vi "一体站流程自动启动.vi"(11 "参数":T1) -> ()   [LabVIEW 2016, in "PLC.lvlib"]
uses:
  PLC.lvlib
panel:
  out "s? t:f":enum16{"初始化", "采配水启动", "仪器操作", "反冲洗", "结束"}(ring)
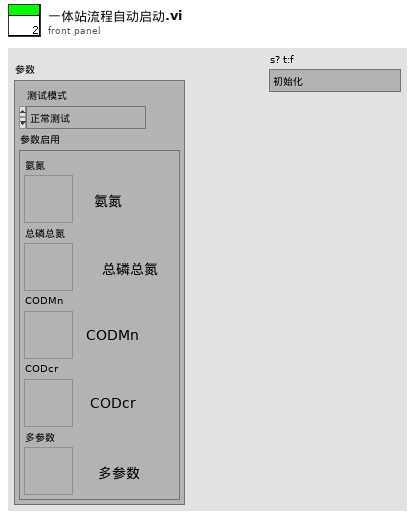
[diagram p1: front panel]
types:
  T1 = cluster{"测试模式":enum16{"正常测试", "集成干预"}, "参数启用":cluster{"氨氮":bool, "总磷总氮":bool, "CODMn":bool, "CODcr":bool, "多参数":bool}}
  T2 = cluster{"命令":string, cluster{"starting address":u16, "holding register value":u16}}
  T3 = enum16{"启动测量", "标样核查", "零点核查", "跨度核查", "空白测试", "平行样测试", "加标回收", "空白校准", "标样校准", "初始化（清洗）", "停止测试", "仪器重启", "校时", "模式设置", "测量间隔设置"}
  T4 = cluster{"时间标识":timestamp, "设备":string, "日志信息":string, "流程参数":string}
  T5 = cluster{"测量模式":enum16{"水样测量", "标样核查", "零点核查", "跨度核查", "空白测试", "加标回收", "平行样", "校零", "校标"}}
  T6 = cluster{"时间标识":timestamp, "设备":string, "日志信息":string}
  T7 = enum16{"空闲", "水样测试", "标样核查", "零点核查", "跨度核查", "空白测试", "平行样测试", "加标回收", "空白校准", "标样校准", "初始化（清洗）"}
  T8 = cluster{"测试时间":dbl, "运行模式":enum16{"维护模式", "常规模式", "应急模式", "质控模式"}}
  T9 = cluster{"R0":i16, "R1":i16, "R2":i16, "R3":i16, "R4":i16, "R5":i16, "R6":i16, "R7":i16, "R8":i16, "R9":i16, "R10":i16, "R11":i16, "R12":i16, "R13":i16, "R14":i16, "R15":i16, "R16":i16, "R17":i16, "R18":i16, "R19":i16, "R20":i16, "R21":i16, "R22":i16, "R23":i16, "R24":i16, "R25":i16, "R26":i16, "R27":i16, "R28":i16, "R29":i16, "R30":i16, "R31":i16, "R32":i16, "R33":i16, "R34":i16}
  T10 = enum32{"Bad", "Idle", "Run top level", "Running"}
  T11 = cluster{"氨氮":bool, "总磷总氮":bool, "CODMn":bool, "CODcr":bool, "多参数":bool}
  T12 = cluster{"水温":dbl, "pH":dbl, "DO":dbl, "Cond":dbl, "Turb":dbl, "叶绿素":dbl, "藻密度":dbl, "蓝绿藻":dbl, "ORP":dbl, "NH3N":dbl}
  T13 = cluster{"时间标识":timestamp, "参数":string, "集成干预测试浓度值":dbl, "集成干预前测试时间":timestamp, "集成干预前测试浓度值":dbl}
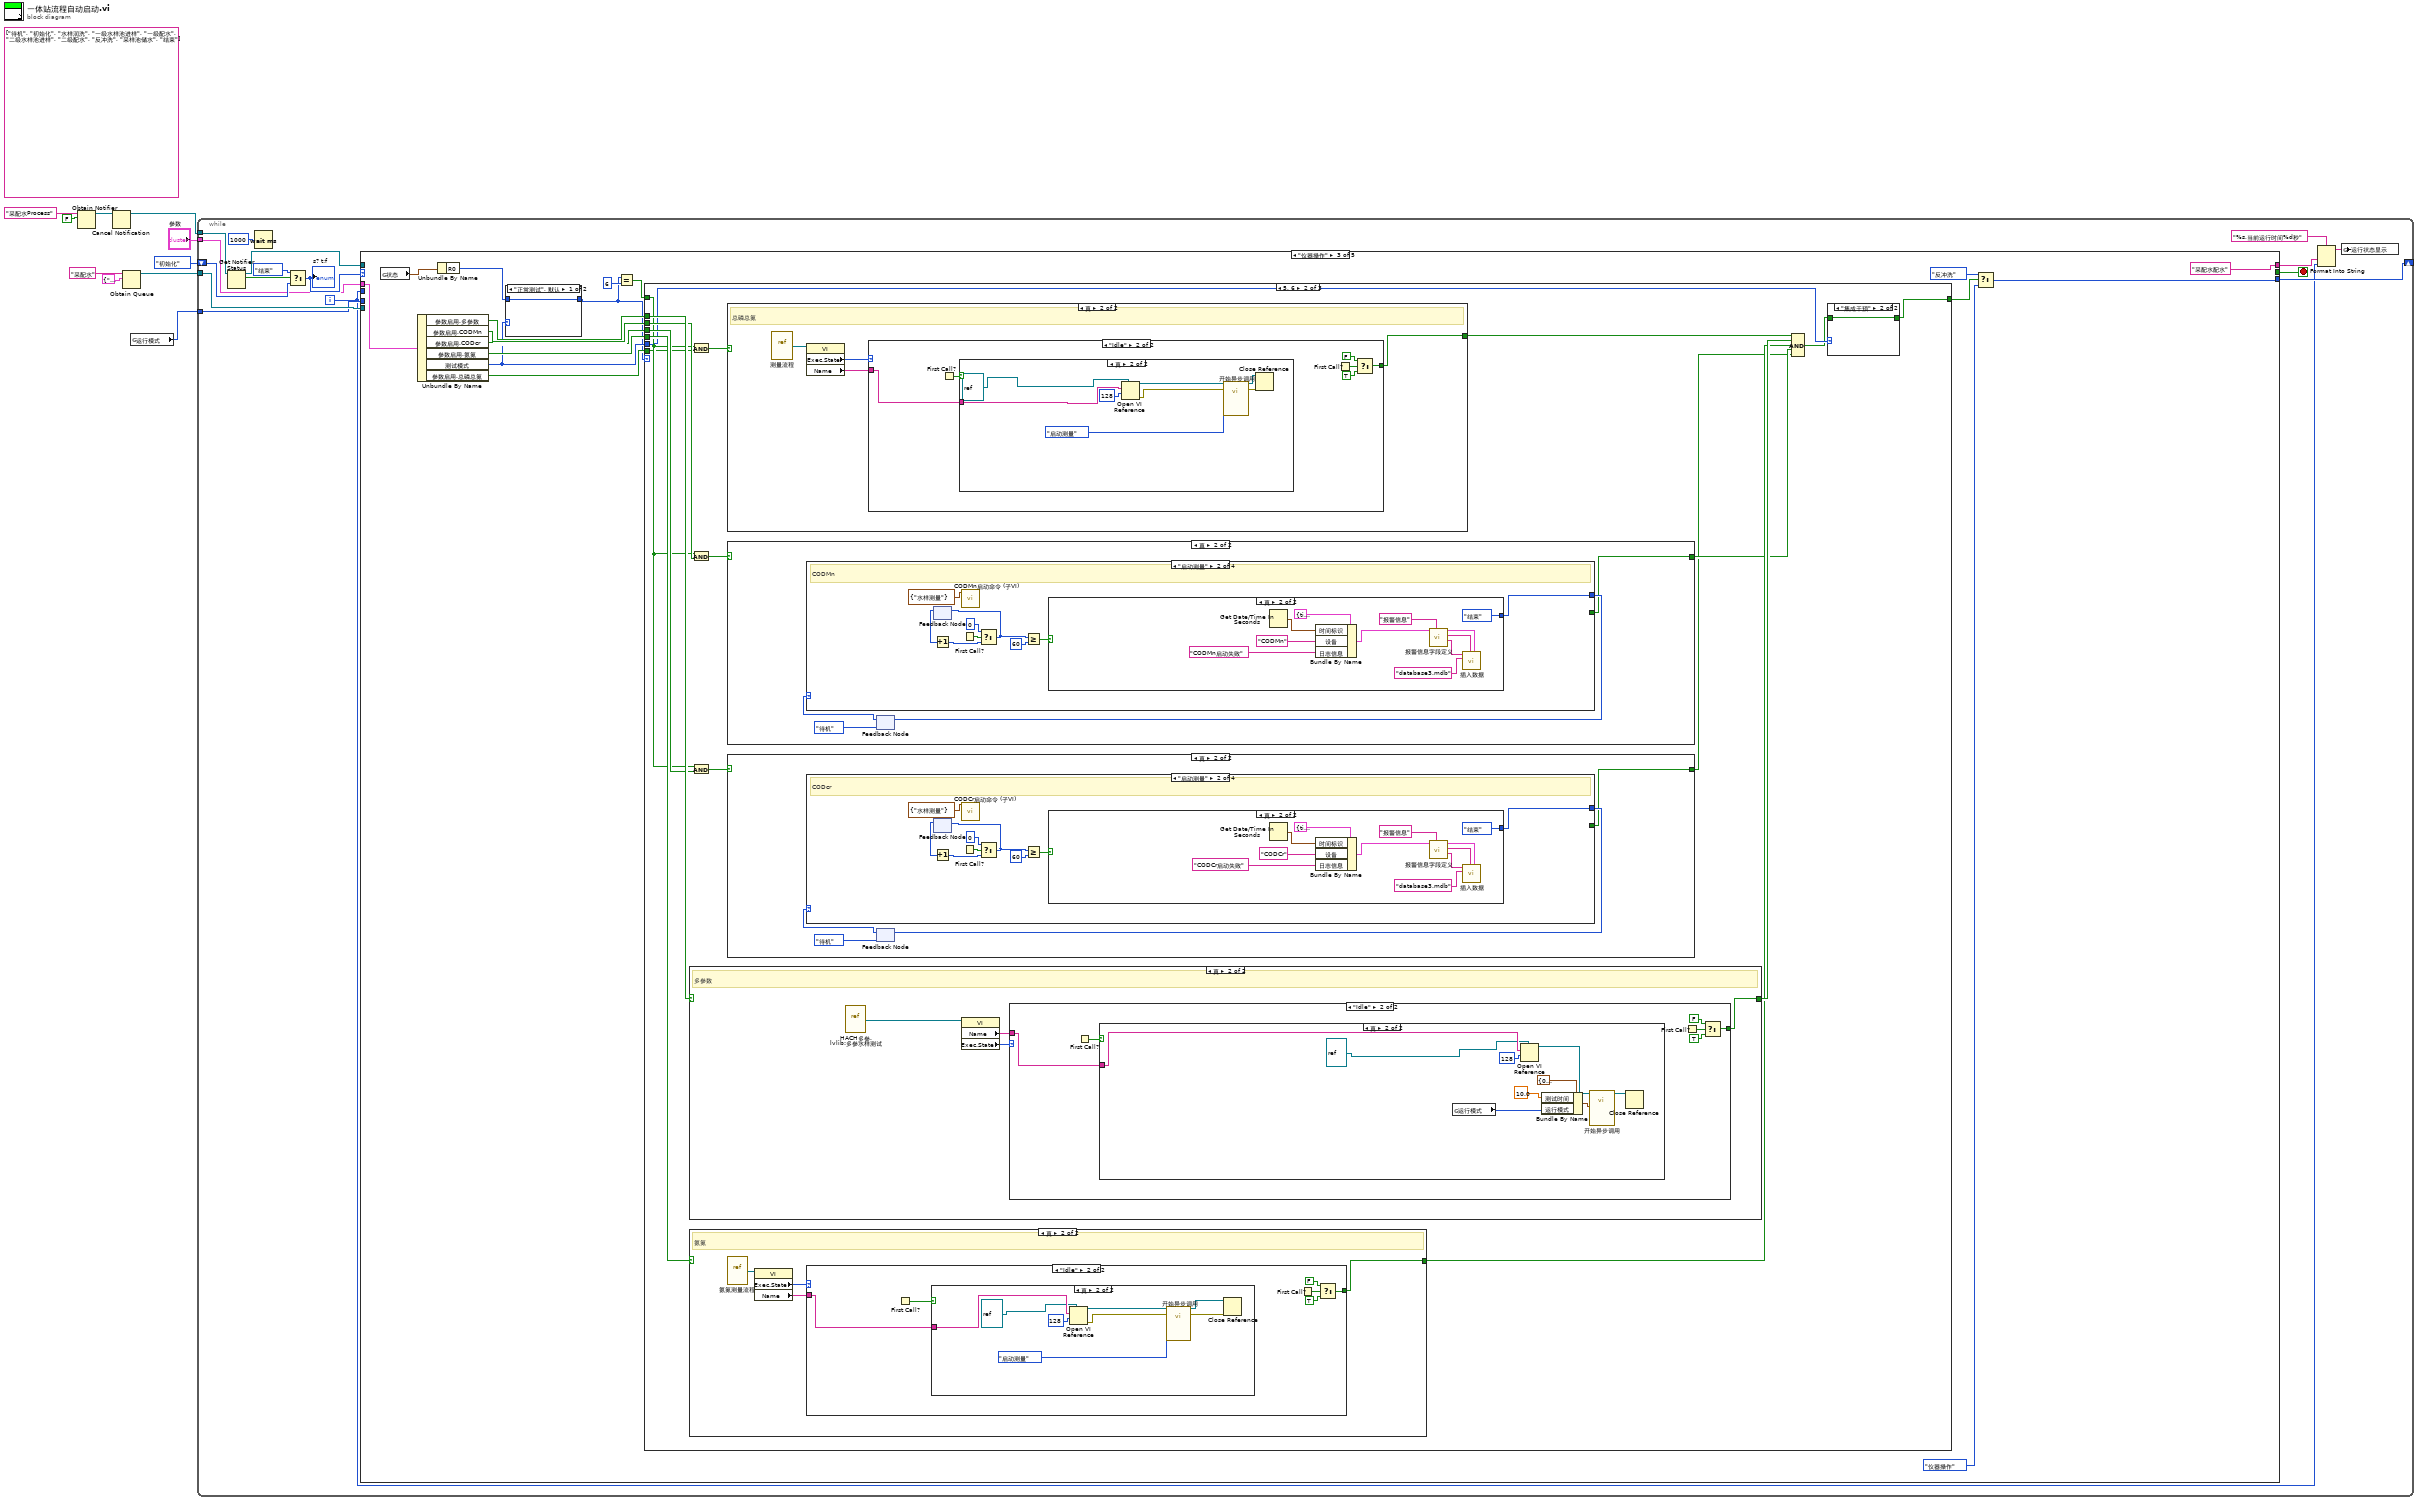
[diagram p0: block diagram]
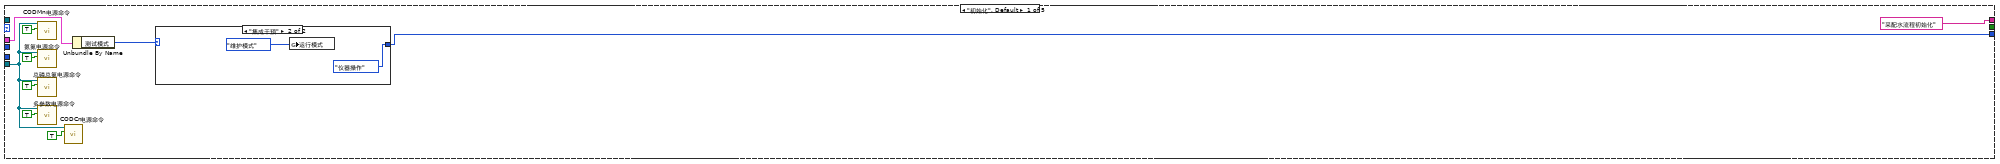
[diagram p2: hidden frame]
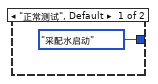
[diagram p3: hidden frame]
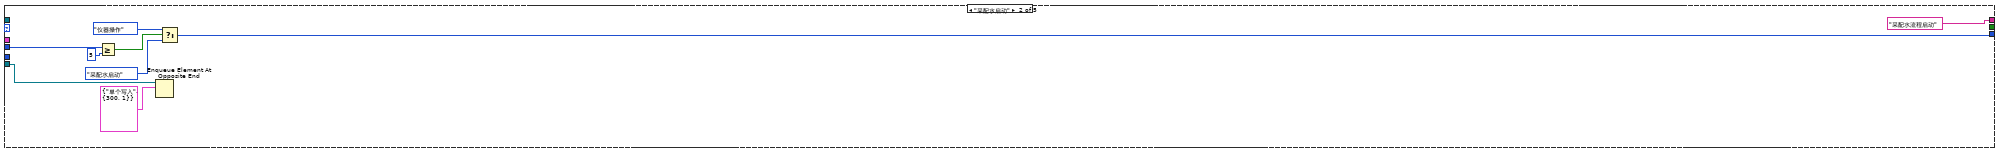
[diagram p4: hidden frame]
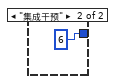
[diagram p5: hidden frame]
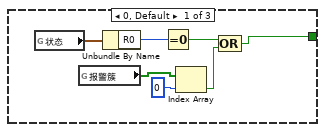
[diagram p6: hidden frame]
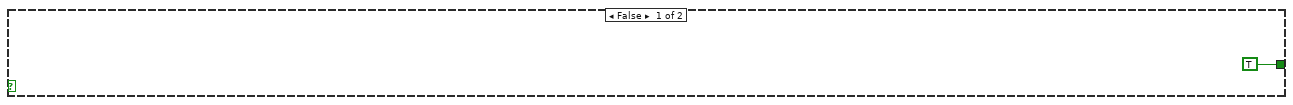
[diagram p7: hidden frame]
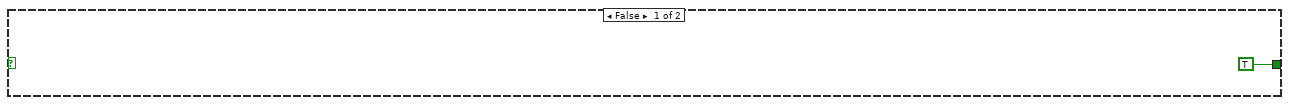
[diagram p11: hidden frame]
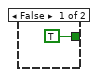
[diagram p14: hidden frame]
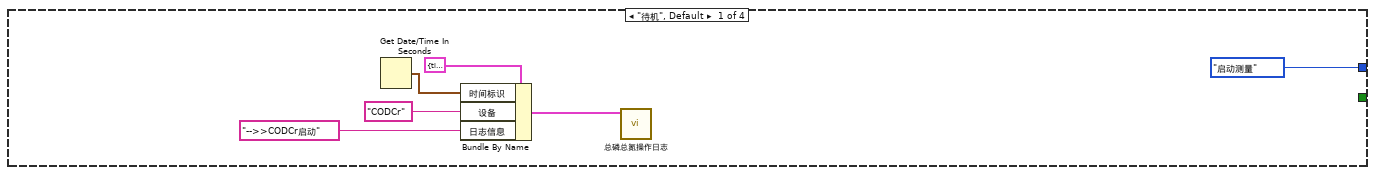
[diagram p15: hidden frame]
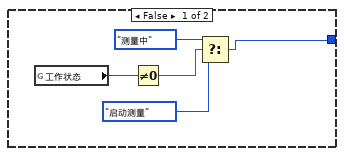
[diagram p16: hidden frame]
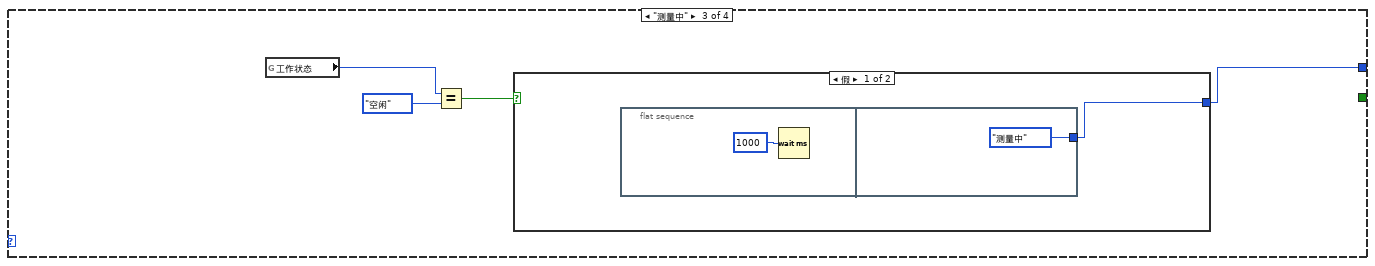
[diagram p17: hidden frame]
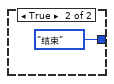
[diagram p18: hidden frame]
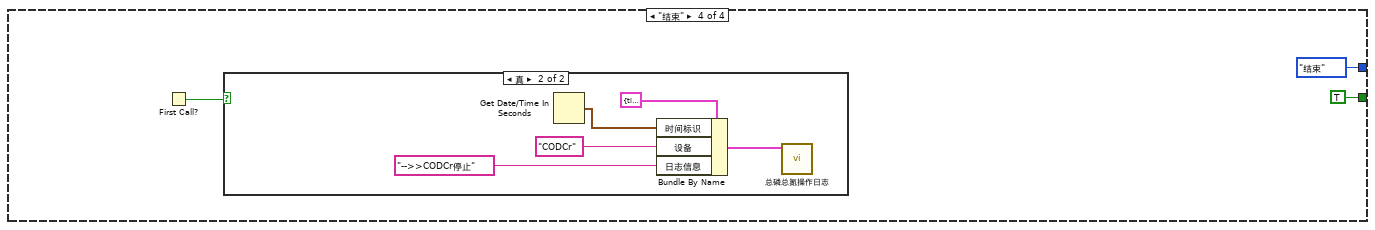
[diagram p19: hidden frame]
diagram:
  (unwired) string[][] [["待机"], ["初始化"], ["水样润洗"], ["一级水样池进样"], ["一级配水"], ["二级水样池进样"], ["二级配水"], ["反冲洗"], ["采样池储水"], ["结束"]] ("项名")
  n1 = Obtain Notifier(name (unnamed)="采配水Process" ("名称（未命名）"), notification data type=FALSE) -> (notifier out=w4:refnum<notifier>)  [unwired: 2 in, 2 out]
  n2 = Cancel Notification(0:w4) -> (8:w3:refnum<notifier>)  [unwired: 1 in, 2 out]
  n3 = Obtain Queue(name (unnamed)="采配水" ("名称（未命名）"), element data type=cluster{"命令":string, "数据":variant} {"命令"="", "数据"=variant}) -> (queue out=w7:refnum<queue>)  [unwired: 3 in, 2 out]
  n4 = global read "系统设置全局变量.vi" "运行模式"() -> (w1:enum16{"维护模式", "常规模式", "应急模式", "质控模式"})
  n5 = while {
    shift-right: [w23] -> _
    shift-left: enum16{"初始化", "采配水启动", "仪器操作", "反冲洗", "结束"}."初始化" ("枚举") -> [w19]
    tunnel: w7 -> [w26]
    tunnel: w3 -> [w22]
    tunnel: "参数" -> [w13]
    tunnel: w1 -> [w12]
    i -> [w11]
    stop <- w25 stop-if-true
    n6 = Get Notifier Status(notifier=w22) -> (notifier out=w14:refnum<notifier>, current notification=w21:bool)  [unwired: 1 in, 3 out]
    n7 = Wait (ms)(milliseconds to wait=u32 1000 ("等待时间（毫秒）")) -> ()  [unwired: 1 out]
    n8 = Select(t=enum16{"初始化", "采配水启动", "仪器操作", "反冲洗", "结束"}."结束" ("枚举"), s=w21, f=w19) -> (s? t:f=w18:enum16{"初始化", "采配水启动", "仪器操作", "反冲洗", "结束"})
    "s? t:f" <- w18
    n9 = case shown="\"仪器操作\"" w18 {
      tunnel: w26 -> [w31 w48 _ _ w434]
      tunnel: [_ _ _ _ TRUE] -> w25
      tunnel: [w30 w40 w60 w258 enum16{"初始化", "采配水启动", "仪器操作", "反冲洗", "结束"}."结束" ("枚举")] -> w23
      tunnel: ["采配水流程初始化" "采配水流程启动" "采配水配水" "等待测试完成" "采配水结束"] -> w15
      tunnel: w14 -> [_ _ _ _ w435]
      tunnel: w13 -> [w28 _ w63 w257 w431]
      tunnel: w12 -> [_ _ _ _ w430]
      tunnel: w11 -> [_ w46 _ _ _]
      frame "初始化", Default {
        n10 = call "CODMn电源命令.vi"("通电/断电"=TRUE, "队列"=w31) -> ()  [unwired: 9 in, 1 out]
        n11 = call "氨氮电源命令.vi"("通电/断电"=TRUE, "队列"=w31) -> ()  [unwired: 9 in, 1 out]
        n12 = call "总磷总氮电源命令.vi"("通电/断电"=TRUE, "队列"=w31) -> ()  [unwired: 9 in, 1 out]
        n13 = call "多参数电源命令.vi"("通电/断电"=TRUE, "队列"=w31) -> ()  [unwired: 9 in, 1 out]
        n14 = call "CODCr电源命令.vi"("通电/断电"=TRUE, "队列"=w31) -> ()  [unwired: 9 in, 1 out]
        n15 = Unbundle By Name(w28) -> ("测试模式"=w27:enum16{"正常测试", "集成干预"})
        n16 = case shown="\"集成干预\"" w27 {
          tunnel: [enum16{"初始化", "采配水启动", "仪器操作", "反冲洗", "结束"}."采配水启动" ("枚举") enum16{"初始化", "采配水启动", "仪器操作", "反冲洗", "结束"}."仪器操作" ("枚举")] -> w30
          frame "正常测试", Default {
          }
          frame "集成干预" {
            n17 = global write "系统设置全局变量.vi" "运行模式"(enum16{"维护模式", "常规模式", "应急模式", "质控模式"}."维护模式" ("运行模式")) -> ()
          }
        }
      }
      frame "采配水启动" {
        n18 = Greater Or Equal?(x=w46, y=5) -> (x >= y?=w43:bool)
        n19 = Enqueue Element At Opposite End(queue=w48, element=T2 {"命令"="单个写入", {"starting address"=300, "holding register value"=1}} ("元素")) -> ()  [unwired: 2 in, 3 out]
        n20 = Select(t=enum16{"初始化", "采配水启动", "仪器操作", "反冲洗", "结束"}."仪器操作" ("枚举"), s=w43, f=enum16{"初始化", "采配水启动", "仪器操作", "反冲洗", "结束"}."采配水启动" ("枚举")) -> (s? t:f=w40:enum16{"初始化", "采配水启动", "仪器操作", "反冲洗", "结束"})
      }
      frame "仪器操作" {
        n21 = global read "采配水全局变量.vi" "状态"() -> (w65:T9)
        n22 = Unbundle By Name(w63) -> ("参数启用.多参数"=w58:bool, "参数启用.CODMn"=w57:bool, "参数启用.CODcr"=w56:bool, "参数启用.氨氮"=w55:bool, "测试模式"=w53:enum16{"正常测试", "集成干预"}, "参数启用.总磷总氮"=w52:bool)
        n23 = Unbundle By Name(w65) -> ("R0"=w54:i16)
        n24 = case shown="\"正常测试\", 默认" w53 {
          tunnel: w54 -> [w66 _]
          tunnel: [w66 i16 6 ("R0")] -> w50
          frame "正常测试", Default {
          }
          frame "集成干预" {
          }
        }
        n25 = Equal?(x=w50, y=i16 6) -> (x = y?=w49:bool)
        n26 = case shown="5, 6" w50 {
          tunnel: [w69 w79 TRUE] -> w62
          tunnel: w58 -> [_ w91 _]
          tunnel: w57 -> [_ w90 _]
          tunnel: w56 -> [_ w87 _]
          tunnel: w55 -> [_ w86 _]
          tunnel: w49 -> [_ w78 _]
          tunnel: w53 -> [_ w81 _]
          tunnel: w52 -> [_ w77 _]
          frame 0, Default {
            n27 = global read "采配水全局变量.vi" "状态"() -> (w72:T9)
            n28 = global read "采配水全局变量.vi" "报警簇"() -> (w73:bool[])
            n29 = Unbundle By Name(w72) -> ("R0"=w71:i16)
            n30 = Equal To 0?(x=w71) -> (x = 0?=w74:bool)
            n31 = Index Array(array=w73, index=0 ("索引")) -> (element=w68:bool)
            n32 = Compound Arithmetic op=OR ("复合运算")(w74, w68) -> (w69:bool)
          }
          frame 5, 6 {
            n33 = case shown="真" w91 {
              tunnel: [TRUE ("t") w235] -> w85
              frame False {
              }
              frame True {
                # "多参数"
                n34 = vi-ref "HACH多参.lvlib:多参水样测试.vi"() -> (w237:refnum<vi>)
                n35 = property class="VI"(reference=w237) -> ("Name"=w236:string, "Exec.State"=w238:T10)  [unwired: 1 in, 2 out]
                n36 = case shown="\"Idle\"" w238 {
                  tunnel: w236 -> [_ w244]
                  tunnel: [_ w239] -> w235
                  frame "Bad", Default {
                  }
                  frame "Idle" {
                    n37 = First Call?() -> (First Call?: T/F=w243:bool)
                    n38 = case shown="真" w243 {
                      tunnel: w244 -> [_ w252]
                      frame False {
                      }
                      frame True {
                        n39 = global read "系统设置全局变量.vi" "运行模式"() -> (w245:enum16{"维护模式", "常规模式", "应急模式", "质控模式"})
                        n40 = Open VI Reference(type specifier VI Refnum (for type only)=refnum<vi> refnum, vi path=w252, options=128 ("选项")) -> (vi reference=w251:refnum<vi>)  [unwired: 3 in, 1 out]
                        n41 = Bundle By Name(cluster=T8 {"测试时间"=0.0, "运行模式"=enum."维护模式"} ("API"), "测试时间"=10.0 ("测量时间"), "运行模式"=w245) -> (w247:T8)
                        n42 = call-by-ref "开始异步调用"(reference=w251, "API"=w247) -> (reference out=w250:refnum<vi>)  [unwired: 12 in, 1 out]
                        n43 = Close Reference(reference=w250) -> ()  [unwired: 1 in, 1 out]
                      }
                    }
                    n44 = First Call?() -> (First Call?: T/F=w242:bool)
                    n45 = Select(t=FALSE, s=w242, f=TRUE) -> (s? t:f=w239:bool)
                  }
                }
              }
            }
            n46 = case "条件结构" shown="真" w86 {
              tunnel: [TRUE ("t") w113] -> w84
              frame False {
              }
              frame True {
                # "氨氮"
                n47 = vi-ref "氨氮测量流程.vi"() -> (w116:refnum<vi>)
                n48 = property class="VI"(reference=w116) -> ("Exec.State"=w115:T10, "Name"=w114:string)  [unwired: 1 in, 2 out]
                n49 = case shown="\"Idle\"" w115 {
                  tunnel: w114 -> [_ w122]
                  tunnel: [_ w117] -> w113
                  frame "Bad", Default {
                  }
                  frame "Idle" {
                    n50 = First Call?() -> (First Call?: T/F=w121:bool)
                    n51 = case shown="真" w121 {
                      tunnel: w122 -> [_ w127]
                      frame False {
                      }
                      frame True {
                        n52 = Open VI Reference(type specifier VI Refnum (for type only)=refnum<vi> refnum, vi path=w127, options=128 ("选项")) -> (vi reference=w125:refnum<vi>, error out=w128:errorcluster)  [unwired: 3 in]
                        n53 = call-by-ref "开始异步调用"(reference=w125, error in=w128, "控制命令"=T3."启动测量") -> (reference out=w129:refnum<vi>, error out=w130:errorcluster)  [unwired: 11 in]
                        n54 = Close Reference(reference=w129, error in (no error)=w130) -> ()  [unwired: 1 out]
                      }
                    }
                    n55 = First Call?() -> (First Call?: T/F=w120:bool)
                    n56 = Select(t=FALSE, s=w120, f=TRUE) -> (s? t:f=w117:bool)
                  }
                }
              }
            }
            n57 = And(x=w78, y=w77) -> (x .and. y?=w76:bool)
            n58 = And(x=w78, y=w90) -> (x .and. y?=w89:bool)
            n59 = And(x=w78, y=w87) -> (x .and. y?=w88:bool)
            n60 = case "条件结构" shown="真" w76 {
              tunnel: [TRUE ("t") w93] -> w75
              frame False {
              }
              frame True {
                # "总磷总氮"
                n61 = vi-ref "测量流程.vi"() -> (w96:refnum<vi>)
                n62 = property class="VI"(reference=w96) -> ("Exec.State"=w95:T10, "Name"=w94:string)  [unwired: 1 in, 2 out]
                n63 = case shown="\"Idle\"" w95 {
                  tunnel: w94 -> [_ w102]
                  tunnel: [_ w97] -> w93
                  frame "Bad", Default {
                  }
                  frame "Idle" {
                    n64 = First Call?() -> (First Call?: T/F=w101:bool)
                    n65 = case shown="真" w101 {
                      tunnel: w102 -> [_ w107]
                      frame False {
                      }
                      frame True {
                        n66 = Open VI Reference(type specifier VI Refnum (for type only)=refnum<vi> refnum, vi path=w107, options=128 ("选项")) -> (vi reference=w105:refnum<vi>, error out=w108:errorcluster)  [unwired: 3 in]
                        n67 = call-by-ref "开始异步调用"(reference=w105, error in=w108, "控制命令"=T3."启动测量") -> (reference out=w109:refnum<vi>, error out=w110:errorcluster)  [unwired: 11 in]
                        n68 = Close Reference(reference=w109, error in (no error)=w110) -> ()  [unwired: 1 out]
                      }
                    }
                    n69 = First Call?() -> (First Call?: T/F=w100:bool)
                    n70 = Select(t=FALSE, s=w100, f=TRUE) -> (s? t:f=w97:bool)
                  }
                }
              }
            }
            n71 = case shown="真" w89 {
              tunnel: [TRUE w184] -> w83
              frame False {
              }
              frame True {
                n72 = feedback #1(enum16{"待机", "启动测量", "测量中", "结束"}."待机") -> (w186:enum16{"待机", "启动测量", "测量中", "结束"})
                n73 = case shown="\"启动测量\"" w186 {
                  tunnel: [enum16{"待机", "启动测量", "测量中", "结束"}."启动测量" w202 w221 enum16{"待机", "启动测量", "测量中", "结束"}."结束"] -> w185
                  tunnel: [_ _ _ TRUE] -> w184
                  frame "待机", Default {
                    n74 = Get Date/Time In Seconds() -> (seconds since 1Jan1904=w192:timestamp)
                    n75 = Bundle By Name(cluster=T4 {"时间标识"=timestamp(0 s since 1904-01-01), "设备"="", "日志信息"="", "流程参数"=""} ("data in"), "时间标识"=w192, "设备"="CODMn", "日志信息"="-->>CODMn启动") -> (w188:T4)
                    n76 = call "总磷总氮操作日志.vi"("data in"=w188) -> ()  [unwired: 11 in]
                  }
                  frame "启动测量" {
                    # "CODMn"
                    n77 = feedback #2() -> (w198:i32)  [unwired: 1 in]
                    n78 = Increment(x=w198) -> (x+1=w199:i32)
                    n79 = First Call?() -> (First Call?: T/F=w197:bool)
                    n80 = call "CODMn启动命令 (子VI).vi"("启动测量模式"=T5 {"测量模式"=enum."水样测量"}) -> ()  [unwired: 11 in]
                    n81 = Select(t=0, s=w197, f=w199) -> (s? t:f=w200:i32)
                    n82 = feedback-in #2(w200) -> ()
                    n83 = Greater Or Equal?(x=w200, y=60) -> (x >= y?=w195:bool)
                    n84 = case shown="真" w195 {
                      tunnel: [w204 enum16{"待机", "启动测量", "测量中", "结束"}."结束"] -> w202
                      frame False {
                        n85 = global read "运行时序全局变量.vi" "多列列表框"() -> (w203:i32)
                        n86 = Not Equal To 0?(x=w203) -> (x != 0?=w205:bool)
                        n87 = Select(t=enum16{"待机", "启动测量", "测量中", "结束"}."测量中", s=w205, f=enum16{"待机", "启动测量", "测量中", "结束"}."启动测量") -> (s? t:f=w204:enum16{"待机", "启动测量", "测量中", "结束"})
                      }
                      frame True {
                        n88 = Get Date/Time In Seconds() -> (seconds since 1Jan1904=w214:timestamp)
                        n89 = Bundle By Name(cluster=T6 {"时间标识"=timestamp(0 s since 1904-01-01), "设备"="", "日志信息"=""} ("data in"), "时间标识"=w214, "设备"="CODMn", "日志信息"="CODMn启动失败") -> (w208:T6)
                        n90 = call "报警信息字段定义.vi"("table输入"="报警信息", "data in"=w208) -> ("table输出"=w211:string, "columns"=w212:string[], "data out"=w213:T6)  [unwired: 7 in]
                        n91 = call "插入数据.vi"("data"=w213, "columns"=w212, "database"="database3.mdb", "table"=w211) -> ()  [unwired: 7 in, 1 out]
                      }
                    }
                  }
                  frame "测量中" {
                    n92 = global read "运行时序全局变量.vi" "多列列表框"() -> (w220:i32)
                    n93 = Equal To 0?(x=w220) -> (x = 0?=w219:bool)
                    n94 = case shown="假" w219 {
                      tunnel: [w222 enum16{"待机", "启动测量", "测量中", "结束"}."结束"] -> w221
                      frame False {
                        n95 = flat-sequence {
                          tunnel: [enum16{"待机", "启动测量", "测量中", "结束"}."测量中"] -> w222
                          frame #0 {
                            n96 = Wait (ms)(milliseconds to wait=u32 1000 ("等待时间（毫秒）")) -> ()  [unwired: 1 out]
                          }
                          frame #1 {
                          }
                        }
                      }
                      frame True {
                      }
                    }
                  }
                  frame "结束" {
                    n97 = First Call?() -> (First Call?: T/F=w226:bool)
                    n98 = case shown="真" w226 {
                      frame False {
                      }
                      frame True {
                        n99 = Get Date/Time In Seconds() -> (seconds since 1Jan1904=w233:timestamp)
                        n100 = Bundle By Name(cluster=T4 {"时间标识"=timestamp(0 s since 1904-01-01), "设备"="", "日志信息"="", "流程参数"=""} ("data in"), "时间标识"=w233, "设备"="CODMn", "日志信息"="-->>CODMn停止") -> (w229:T4)
                        n101 = call "总磷总氮操作日志.vi"("data in"=w229) -> ()  [unwired: 11 in]
                      }
                    }
                  }
                }
                n102 = feedback-in #1(w185) -> ()
              }
            }
            n103 = case shown="真" w88 {
              tunnel: [TRUE w132] -> w82
              frame False {
              }
              frame True {
                n104 = feedback #3(enum16{"待机", "启动测量", "测量中", "结束"}."待机") -> (w134:enum16{"待机", "启动测量", "测量中", "结束"})
                n105 = case shown="\"启动测量\"" w134 {
                  tunnel: [enum16{"待机", "启动测量", "测量中", "结束"}."启动测量" w150 w170 enum16{"待机", "启动测量", "测量中", "结束"}."结束"] -> w133
                  tunnel: [_ _ _ TRUE] -> w132
                  frame "待机", Default {
                    n106 = Get Date/Time In Seconds() -> (seconds since 1Jan1904=w140:timestamp)
                    n107 = Bundle By Name(cluster=T4 {"时间标识"=timestamp(0 s since 1904-01-01), "设备"="", "日志信息"="", "流程参数"=""} ("data in"), "时间标识"=w140, "设备"="CODCr", "日志信息"="-->>CODCr启动") -> (w136:T4)
                    n108 = call "总磷总氮操作日志.vi"("data in"=w136) -> ()  [unwired: 11 in]
                  }
                  frame "启动测量" {
                    # "CODcr"
                    n109 = feedback #4() -> (w146:i32)  [unwired: 1 in]
                    n110 = Increment(x=w146) -> (x+1=w147:i32)
                    n111 = First Call?() -> (First Call?: T/F=w145:bool)
                    n112 = call "CODCr启动命令 (子VI).vi"("启动测量模式"=T5 {"测量模式"=enum."水样测量"}) -> ()  [unwired: 11 in]
                    n113 = Select(t=0, s=w145, f=w147) -> (s? t:f=w148:i32)
                    n114 = feedback-in #4(w148) -> ()
                    n115 = Greater Or Equal?(x=w148, y=60) -> (x >= y?=w143:bool)
                    n116 = case shown="真" w143 {
                      tunnel: [w151 enum16{"待机", "启动测量", "测量中", "结束"}."结束"] -> w150
                      frame False {
                        n117 = global read "CODcr全局变量.vi" "工作状态"() -> (w152:T7)
                        n118 = Not Equal To 0?(x=w152) -> (x != 0?=w153:bool)
                        n119 = Select(t=enum16{"待机", "启动测量", "测量中", "结束"}."测量中", s=w153, f=enum16{"待机", "启动测量", "测量中", "结束"}."启动测量") -> (s? t:f=w151:enum16{"待机", "启动测量", "测量中", "结束"})
                      }
                      frame True {
                        n120 = Get Date/Time In Seconds() -> (seconds since 1Jan1904=w162:timestamp)
                        n121 = Bundle By Name(cluster=T6 {"时间标识"=timestamp(0 s since 1904-01-01), "设备"="", "日志信息"=""} ("data in"), "时间标识"=w162, "设备"="CODCr", "日志信息"="CODCr启动失败") -> (w156:T6)
                        n122 = call "报警信息字段定义.vi"("table输入"="报警信息", "data in"=w156) -> ("table输出"=w159:string, "columns"=w160:string[], "data out"=w161:T6)  [unwired: 7 in]
                        n123 = call "插入数据.vi"("data"=w161, "columns"=w160, "database"="database3.mdb", "table"=w159) -> ()  [unwired: 7 in, 1 out]
                      }
                    }
                  }
                  frame "测量中" {
                    n124 = global read "CODcr全局变量.vi" "工作状态"() -> (w169:T7)
                    n125 = Equal?(x=w169, y=T7."空闲" ("工作状态")) -> (x = y?=w168:bool)
                    n126 = case shown="假" w168 {
                      tunnel: [w171 enum16{"待机", "启动测量", "测量中", "结束"}."结束"] -> w170
                      frame False {
                        n127 = flat-sequence {
                          tunnel: [enum16{"待机", "启动测量", "测量中", "结束"}."测量中"] -> w171
                          frame #0 {
                            n128 = Wait (ms)(milliseconds to wait=u32 1000 ("等待时间（毫秒）")) -> ()  [unwired: 1 out]
                          }
                          frame #1 {
                          }
                        }
                      }
                      frame True {
                      }
                    }
                  }
                  frame "结束" {
                    n129 = First Call?() -> (First Call?: T/F=w175:bool)
                    n130 = case shown="真" w175 {
                      frame False {
                      }
                      frame True {
                        n131 = Get Date/Time In Seconds() -> (seconds since 1Jan1904=w182:timestamp)
                        n132 = Bundle By Name(cluster=T4 {"时间标识"=timestamp(0 s since 1904-01-01), "设备"="", "日志信息"="", "流程参数"=""} ("data in"), "时间标识"=w182, "设备"="CODCr", "日志信息"="-->>CODCr停止") -> (w178:T4)
                        n133 = call "总磷总氮操作日志.vi"("data in"=w178) -> ()  [unwired: 11 in]
                      }
                    }
                  }
                }
                n134 = feedback-in #3(w133) -> ()
              }
            }
            n135 = Compound Arithmetic op=AND ("复合运算")(w75, w85, w84, w83, w82) -> (w80:bool)
            n136 = case shown="\"集成干预\"" w81 {
              tunnel: w80 -> [_ w111]
              tunnel: [_ w111] -> w79
              frame "正常测试", Default {
              }
              frame "集成干预" {
              }
            }
          }
          frame 7..9 {
          }
        }
        n137 = Select(t=enum16{"初始化", "采配水启动", "仪器操作", "反冲洗", "结束"}."反冲洗" ("枚举"), s=w62, f=enum16{"初始化", "采配水启动", "仪器操作", "反冲洗", "结束"}."仪器操作" ("枚举")) -> (s? t:f=w60:enum16{"初始化", "采配水启动", "仪器操作", "反冲洗", "结束"})
      }
      frame "反冲洗" {
        n138 = First Call?() -> (First Call?: T/F=w255:bool)
        n139 = case shown="真" w255 {
          tunnel: w257 -> [_ w266]
          frame False {
          }
          frame True {
            n140 = Unbundle By Name(w266) -> ("测试模式"=w265:enum16{"正常测试", "集成干预"}, "参数启用"=w264:T11)
            n141 = case shown="\"正常测试\", 默认" w265 {
              tunnel: w264 -> [w269 w361]
              frame "正常测试", Default {
                n142 = global read "系统设置全局变量.vi" "运行模式"() -> (w267:enum16{"维护模式", "常规模式", "应急模式", "质控模式"})
                n143 = global read "采配水全局变量.vi" "报警簇"() -> (w274:bool[])
                n144 = case shown="\"维护模式\"" w267 {
                  tunnel: ["M" ("table") "N" ("table")] -> w268
                  frame "维护模式" {
                  }
                  frame "常规模式", Default {
                  }
                }
                n145 = Index Array(array=w274, index #1=0 ("索引"), index #2=11 ("索引")) -> (element #1=w271:bool, element #2=w270:bool)
                n146 = case shown="真" w271 {
                  tunnel: w270 -> [w280 _]
                  tunnel: w269 -> [w279 w293]
                  tunnel: w268 -> [w277 w287]
                  frame False {
                    n147 = Unbundle By Name(w279) -> ("氨氮"=w278:bool)
                    n148 = case shown="真" w280 {
                      tunnel: w278 -> [_ w282]
                      tunnel: w277 -> [_ w281]
                      frame False {
                      }
                      frame True {
                        n149 = case shown="真" w282 {
                          tunnel: w281 -> [_ w283]
                          tunnel: [_ w284] -> _
                          frame False {
                          }
                          frame True {
                            n150 = call "取水点无水样数据存储.vi"("数据标识"="lw", "数据类型"=w283, "table"="氨氮") -> ("error out"=w284:errorcluster)  [unwired: 8 in]
                          }
                        }
                      }
                    }
                  }
                  frame True {
                    n151 = Unbundle By Name(w293) -> ("氨氮"=w292:bool, "CODMn"=w291:bool, "CODcr"=w290:bool, "多参数"=w289:bool, "总磷总氮"=w288:bool)
                    n152 = case shown="真" w292 {
                      tunnel: w287 -> [_ w353]
                      tunnel: [_ w354] -> _
                      frame False {
                      }
                      frame True {
                        n153 = call "取水点无水样数据存储.vi"("数据标识"="Z", "数据类型"=w353, "table"="氨氮") -> ("error out"=w354:errorcluster)  [unwired: 8 in]
                      }
                    }
                    n154 = case shown="真" w291 {
                      tunnel: w287 -> [_ w350]
                      tunnel: [_ w349] -> _
                      frame False {
                      }
                      frame True {
                        n155 = call "取水点无水样数据存储.vi"("数据标识"="Z", "数据类型"=w350, "table"="CODMn") -> ("error out"=w349:errorcluster)  [unwired: 8 in]
                      }
                    }
                    n156 = case shown="真" w290 {
                      tunnel: w287 -> [_ w346]
                      tunnel: [_ w345] -> _
                      frame False {
                      }
                      frame True {
                        n157 = call "取水点无水样数据存储.vi"("数据标识"="Z", "数据类型"=w346, "table"="CODCr") -> ("error out"=w345:errorcluster)  [unwired: 8 in]
                      }
                    }
                    n158 = case shown="真" w288 {
                      tunnel: w287 -> [_ w295]
                      tunnel: [_ w294] -> _
                      frame False {
                      }
                      frame True {
                        n159 = call "取水点无水样数据存储.vi"("数据标识"="Z", "数据类型"=w295, "table"="总氮") -> ("error out"=w296:errorcluster)  [unwired: 8 in]
                        n160 = call "取水点无水样数据存储.vi"("error in (no error)"=w296, "数据标识"="Z", "数据类型"=w295, "table"="总磷") -> ("error out"=w294:errorcluster)  [unwired: 7 in]
                      }
                    }
                    n161 = case shown="真" w289 {
                      tunnel: w287 -> [_ w301]
                      frame False {
                      }
                      frame True {
                        n162 = global read "多参数全局变量.vi" "传感器通道号"() -> (w316:T12)
                        n163 = Unbundle By Name(w316) -> ("水温"=w315:dbl, "pH"=w314:dbl, "DO"=w313:dbl, "Cond"=w312:dbl, "Turb"=w311:dbl, "叶绿素"=w310:dbl, "藻密度"=w309:dbl)
                        n164 = Not Equal To 0?(x=w315) -> (x != 0?=w308:bool)
                        n165 = Not Equal To 0?(x=w314) -> (x != 0?=w307:bool)
                        n166 = Not Equal To 0?(x=w313) -> (x != 0?=w306:bool)
                        n167 = Not Equal To 0?(x=w312) -> (x != 0?=w305:bool)
                        n168 = Not Equal To 0?(x=w311) -> (x != 0?=w304:bool)
                        n169 = Not Equal To 0?(x=w310) -> (x != 0?=w303:bool)
                        n170 = Not Equal To 0?(x=w309) -> (x != 0?=w302:bool)
                        n171 = case shown="真" w308 {
                          tunnel: w301 -> [_ w342]
                          tunnel: [_ w341] -> _
                          frame False {
                          }
                          frame True {
                            n172 = call "取水点无水样数据存储.vi"("数据标识"="Z", "数据类型"=w342, "table"="水温") -> ("error out"=w341:errorcluster)  [unwired: 8 in]
                          }
                        }
                        n173 = case shown="真" w307 {
                          tunnel: w301 -> [_ w338]
                          tunnel: [_ w337] -> _
                          frame False {
                          }
                          frame True {
                            n174 = call "取水点无水样数据存储.vi"("数据标识"="Z", "数据类型"=w338, "table"="pH") -> ("error out"=w337:errorcluster)  [unwired: 8 in]
                          }
                        }
                        n175 = case shown="真" w306 {
                          tunnel: w301 -> [_ w334]
                          tunnel: [_ w333] -> _
                          frame False {
                          }
                          frame True {
                            n176 = call "取水点无水样数据存储.vi"("数据标识"="Z", "数据类型"=w334, "table"="DO") -> ("error out"=w333:errorcluster)  [unwired: 8 in]
                          }
                        }
                        n177 = case shown="真" w304 {
                          tunnel: w301 -> [_ w326]
                          tunnel: [_ w325] -> _
                          frame False {
                          }
                          frame True {
                            n178 = call "取水点无水样数据存储.vi"("数据标识"="Z", "数据类型"=w326, "table"="浊度") -> ("error out"=w325:errorcluster)  [unwired: 8 in]
                          }
                        }
                        n179 = case shown="真" w305 {
                          tunnel: w301 -> [_ w330]
                          tunnel: [_ w329] -> _
                          frame False {
                          }
                          frame True {
                            n180 = call "取水点无水样数据存储.vi"("数据标识"="Z", "数据类型"=w330, "table"="比电导率") -> ("error out"=w329:errorcluster)  [unwired: 8 in]
                          }
                        }
                        n181 = case shown="真" w303 {
                          tunnel: w301 -> [_ w322]
                          tunnel: [_ w321] -> _
                          frame False {
                          }
                          frame True {
                            n182 = call "取水点无水样数据存储.vi"("数据标识"="Z", "数据类型"=w322, "table"="叶绿素") -> ("error out"=w321:errorcluster)  [unwired: 8 in]
                          }
                        }
                        n183 = case shown="真" w302 {
                          tunnel: w301 -> [_ w318]
                          tunnel: [_ w317] -> _
                          frame False {
                          }
                          frame True {
                            n184 = call "取水点无水样数据存储.vi"("数据标识"="Z", "数据类型"=w318, "table"="藻密度") -> ("error out"=w317:errorcluster)  [unwired: 8 in]
                          }
                        }
                      }
                    }
                  }
                }
              }
              frame "集成干预" {
                n185 = Unbundle By Name(w361) -> ("氨氮"=w360:bool, "CODMn"=w359:bool, "CODcr"=w358:bool, "多参数"=w357:bool)
                n186 = case shown="真" w360 {
                  frame False {
                  }
                  frame True {
                    n187 = call "获取最近两组水样测试数据.vi"("table"="氨氮") -> ("error out"=w427:errorcluster, "存储变量"=w428:T13)  [unwired: 9 in]
                    n188 = call "集成干预测试数据存储.vi"("error in (no error)"=w427, "存储变量"=w428) -> ("error out"=w423:errorcluster)  [unwired: 9 in]
                    n189 = call "获取最近两组水样测试数据.vi"("error in (no error)"=w423, "table"="总磷") -> ("error out"=w426:errorcluster, "存储变量"=w425:T13)  [unwired: 8 in]
                    n190 = call "集成干预测试数据存储.vi"("error in (no error)"=w426, "存储变量"=w425) -> ()  [unwired: 9 in, 1 out]
                  }
                }
                n191 = case shown="真" w359 {
                  frame False {
                  }
                  frame True {
                    n192 = call "获取最近两组水样测试数据.vi"("table"="CODMn") -> ("error out"=w420:errorcluster, "存储变量"=w421:T13)  [unwired: 9 in]
                    n193 = call "集成干预测试数据存储.vi"("error in (no error)"=w420, "存储变量"=w421) -> ()  [unwired: 9 in, 1 out]
                  }
                }
                n194 = case shown="真" w358 {
                  frame False {
                  }
                  frame True {
                    n195 = call "获取最近两组水样测试数据.vi"("table"="CODCr") -> ("error out"=w417:errorcluster, "存储变量"=w418:T13)  [unwired: 9 in]
                    n196 = call "集成干预测试数据存储.vi"("error in (no error)"=w417, "存储变量"=w418) -> ()  [unwired: 9 in, 1 out]
                  }
                }
                n197 = case shown="真" w357 {
                  frame False {
                  }
                  frame True {
                    n198 = global read "多参数全局变量.vi" "传感器通道号"() -> (w382:T12)
                    n199 = Unbundle By Name(w382) -> ("水温"=w381:dbl, "pH"=w378:dbl, "DO"=w375:dbl, "Cond"=w372:dbl, "Turb"=w370:dbl, "叶绿素"=w369:dbl, "藻密度"=w368:dbl)
                    n200 = Not Equal To 0?(x=w381) -> (x != 0?=w380:bool)
                    n201 = Not Equal To 0?(x=w378) -> (x != 0?=w377:bool)
                    n202 = case shown="真" w380 {
                      tunnel: [_ w413] -> w379
                      frame False {
                      }
                      frame True {
                        n203 = call "获取最近两组水样测试数据.vi"("table"="水温") -> ("error out"=w416:errorcluster, "存储变量"=w415:T13)  [unwired: 9 in]
                        n204 = call "集成干预测试数据存储.vi"("error in (no error)"=w416, "存储变量"=w415) -> ("error out"=w413:errorcluster)  [unwired: 9 in]
                      }
                    }
                    n205 = Not Equal To 0?(x=w368) -> (x != 0?=w362:bool)
                    n206 = Not Equal To 0?(x=w369) -> (x != 0?=w364:bool)
                    n207 = Not Equal To 0?(x=w370) -> (x != 0?=w366:bool)
                    n208 = Not Equal To 0?(x=w372) -> (x != 0?=w371:bool)
                    n209 = Not Equal To 0?(x=w375) -> (x != 0?=w374:bool)
                    n210 = case shown="真" w377 {
                      tunnel: [_ w409] -> w376
                      tunnel: w379 -> [_ w408]
                      frame False {
                      }
                      frame True {
                        n211 = call "获取最近两组水样测试数据.vi"("error in (no error)"=w408, "table"="pH") -> ("error out"=w412:errorcluster, "存储变量"=w411:T13)  [unwired: 8 in]
                        n212 = call "集成干预测试数据存储.vi"("error in (no error)"=w412, "存储变量"=w411) -> ("error out"=w409:errorcluster)  [unwired: 9 in]
                      }
                    }
                    n213 = case shown="真" w374 {
                      tunnel: [_ w404] -> w373
                      tunnel: w376 -> [_ w403]
                      frame False {
                      }
                      frame True {
                        n214 = call "获取最近两组水样测试数据.vi"("error in (no error)"=w403, "table"="DO") -> ("error out"=w407:errorcluster, "存储变量"=w406:T13)  [unwired: 8 in]
                        n215 = call "集成干预测试数据存储.vi"("error in (no error)"=w407, "存储变量"=w406) -> ("error out"=w404:errorcluster)  [unwired: 9 in]
                      }
                    }
                    n216 = case shown="真" w371 {
                      tunnel: [_ w399] -> w367
                      tunnel: w373 -> [_ w398]
                      frame False {
                      }
                      frame True {
                        n217 = call "获取最近两组水样测试数据.vi"("error in (no error)"=w398, "table"="比电导率") -> ("error out"=w402:errorcluster, "存储变量"=w401:T13)  [unwired: 8 in]
                        n218 = call "集成干预测试数据存储.vi"("error in (no error)"=w402, "存储变量"=w401) -> ("error out"=w399:errorcluster)  [unwired: 9 in]
                      }
                    }
                    n219 = case shown="真" w366 {
                      tunnel: [_ w394] -> w365
                      tunnel: w367 -> [_ w393]
                      frame False {
                      }
                      frame True {
                        n220 = call "获取最近两组水样测试数据.vi"("error in (no error)"=w393, "table"="浊度") -> ("error out"=w397:errorcluster, "存储变量"=w396:T13)  [unwired: 8 in]
                        n221 = call "集成干预测试数据存储.vi"("error in (no error)"=w397, "存储变量"=w396) -> ("error out"=w394:errorcluster)  [unwired: 9 in]
                      }
                    }
                    n222 = case shown="真" w364 {
                      tunnel: [_ w389] -> w363
                      tunnel: w365 -> [_ w388]
                      frame False {
                      }
                      frame True {
                        n223 = call "获取最近两组水样测试数据.vi"("error in (no error)"=w388, "table"="叶绿素") -> ("error out"=w392:errorcluster, "存储变量"=w391:T13)  [unwired: 8 in]
                        n224 = call "集成干预测试数据存储.vi"("error in (no error)"=w392, "存储变量"=w391) -> ("error out"=w389:errorcluster)  [unwired: 9 in]
                      }
                    }
                    n225 = case shown="真" w362 {
                      tunnel: [_ w384] -> _
                      tunnel: w363 -> [_ w383]
                      frame False {
                      }
                      frame True {
                        n226 = call "获取最近两组水样测试数据.vi"("error in (no error)"=w383, "table"="藻密度") -> ("error out"=w387:errorcluster, "存储变量"=w386:T13)  [unwired: 8 in]
                        n227 = call "集成干预测试数据存储.vi"("error in (no error)"=w387, "存储变量"=w386) -> ("error out"=w384:errorcluster)  [unwired: 9 in]
                      }
                    }
                  }
                }
              }
            }
          }
        }
        n228 = global read "采配水全局变量.vi" "状态"() -> (w263:T9)
        n229 = Unbundle By Name(w263) -> ("R0"=w262:i16)
        n230 = Equal To 0?(x=w262) -> (x = 0?=w261:bool)
        n231 = Select(t=enum16{"初始化", "采配水启动", "仪器操作", "反冲洗", "结束"}."结束" ("枚举"), s=w261, f=enum16{"初始化", "采配水启动", "仪器操作", "反冲洗", "结束"}."反冲洗" ("枚举")) -> (s? t:f=w258:enum16{"初始化", "采配水启动", "仪器操作", "反冲洗", "结束"})
      }
      frame "结束" {
        n232 = Release Queue(queue=w434) -> ()  [unwired: 2 in, 3 out]
        n233 = Unbundle By Name(w431) -> ("测试模式"=w432:enum16{"正常测试", "集成干预"})
        n234 = Cancel Notification(0:w435) -> (8:w436:refnum<notifier>)  [unwired: 1 in, 2 out]
        n235 = Release Notifier(notifier=w436) -> ()  [unwired: 2 in, 3 out]
        n236 = case shown="\"集成干预\"" w432 {
          tunnel: w430 -> [_ w439]
          frame "正常测试", Default {
          }
          frame "集成干预" {
            n237 = global write "系统设置全局变量.vi" "运行模式"(w439) -> ()
          }
        }
      }
    }
    n238 = Format Into String(format string="%s,当前运行时间%d秒" ("格式字符串"), w15, w11) -> (resulting string=w16:string)  [unwired: 2 in, 1 out]
    n239 = global write "采配水全局变量.vi" "运行状态显示"(w16) -> ()
  }
